vi "RT Subparse properties.vi"(5 "FIFO Index Decimation Table":i32[](array[numeric])=[0, 2, 2, 0, 3], 7 "Block Address decimation table":u32[](array[numeric])=[0, 2, 2, 0, 3], 8 "FIFO indexes":i32[](array[numeric])=[1, 2, 3, 4, 5], 9 "Block Address":u32[](array[numeric])=[0, 2, 2, 0, 3], 11 "Relative Address in Block":u32[](array[numeric])=[0, 0, 1, 5, 5]) -> (0 "error out":errorcluster, 2 "Array out":T1[](array[typedef]), 3 "max block size":u32)   [LabVIEW 2015, in "RefMem DMA Custom Device.lvlib"]
uses:
  RefMem DMA Custom Device.lvlib
  Block descriptor.ctl
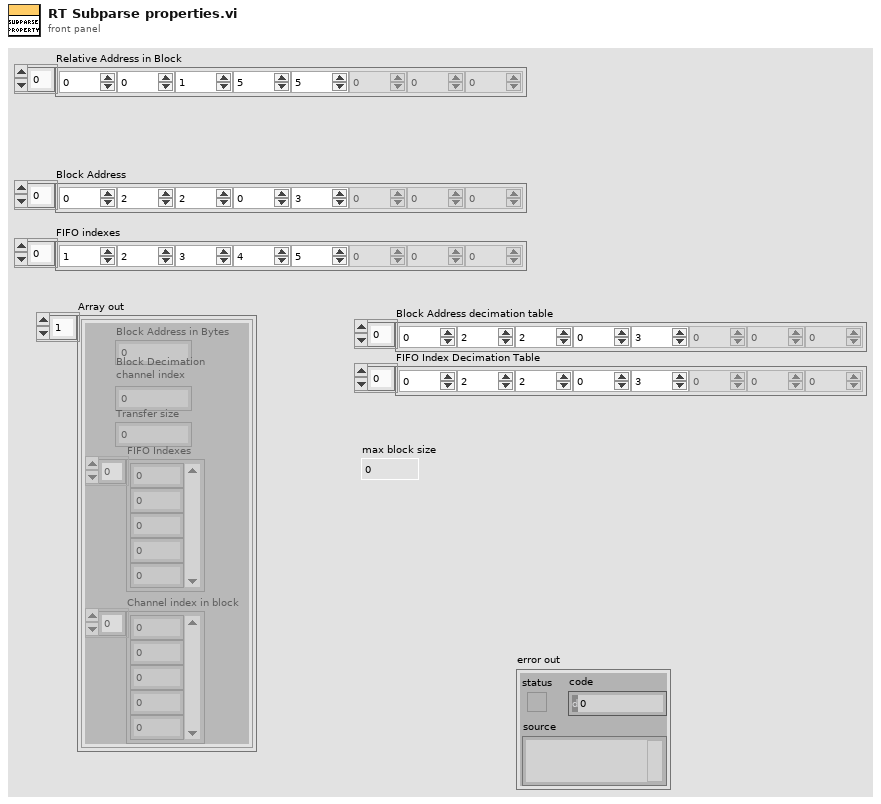
[diagram p1: front panel]
types:
  T1 = typedef "RefMem DMA Custom Device.lvlib/Block descriptor.ctl" = cluster{"Block Address in Bytes":u32, "Block Decimation \nchannel index":i32, "Transfer size":u32, "FIFO Indexes":i32[], "Channel index in block":i32[]}
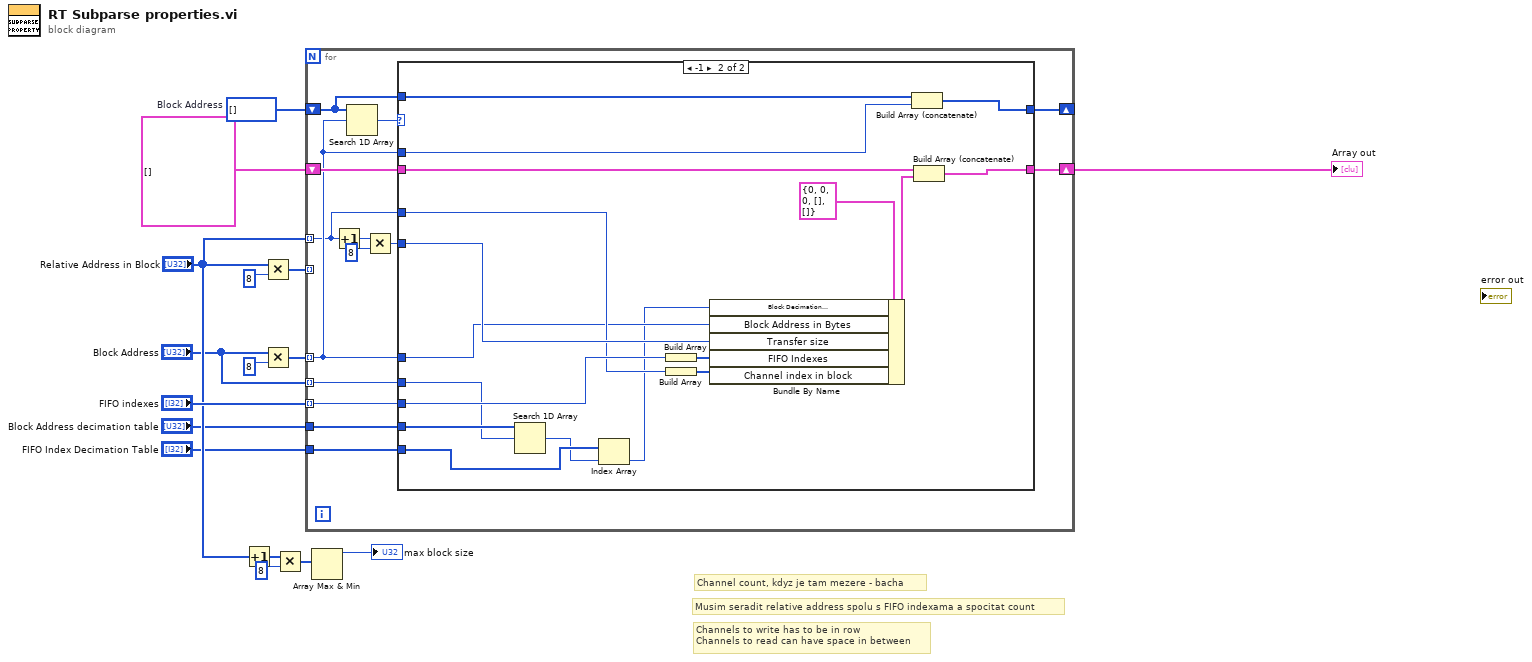
[diagram p0: block diagram]
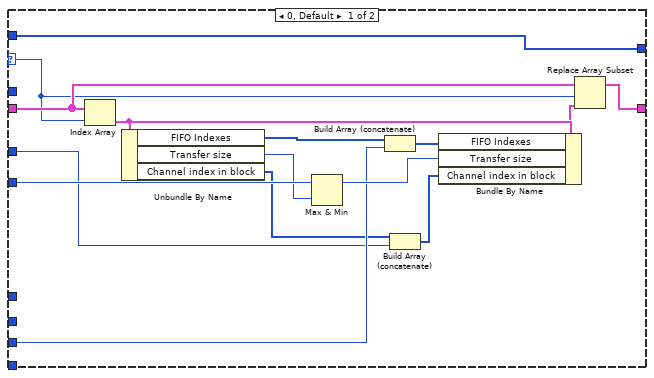
[diagram p2: hidden frame]
diagram:
  w15 = u32[] []  # Block Address
  # "Channel count, kdyz je tam mezere - bacha"
  # "Channels to write has to be in row\nChannels to read can have space in between"
  # "Musim seradit relative address spolu s FIFO indexama a spocitat count"
  n1 = Increment(x="Relative Address in Block") -> (x+1=w6:u32[])
  n2 = Multiply(x="Relative Address in Block", y=u32 8) -> (x*y=w11:u32[])
  n3 = Multiply(x="Block Address", y=u32 8) -> (x*y=w8:u32[])
  n4 = Multiply(x=w6, y=u32 8) -> (x*y=w4:u32[])
  n5 = for {
    tunnel: w8 -> [w25] mode=indexing
    tunnel: "FIFO indexes" -> [w24] mode=indexing
    shift-right: [w27] -> _
    shift-left: w15 -> [w29]
    shift-right: [w26] -> w13
    shift-left: T1[] [] ("Array out") -> [w28]
    tunnel: w11 -> [_] mode=indexing
    tunnel: "Relative Address in Block" -> [w20] mode=indexing
    tunnel: "Block Address decimation table" -> [w19]
    tunnel: "FIFO Index Decimation Table" -> [w18]
    tunnel: "Block Address" -> [w17] mode=indexing
    n6 = Increment(x=w20) -> (x+1=w23:u32)
    n7 = Search 1D Array(1D array=w29, element=w25) -> (index of element=w30:i32)  [unwired: 1 in]
    n8 = Multiply(x=w23, y=u32 8) -> (x*y=w21:u32)
    n9 = case shown="-1" w30 {
      selector: w30 -> [w43 _]
      tunnel: w29 -> [w40 w63]
      tunnel: w28 -> [w44 w62]
      tunnel: [w40 w61] -> w27
      tunnel: [w42 w60] -> w26
      tunnel: w25 -> [_ w59]
      tunnel: w25 -> [_ w50]
      tunnel: w24 -> [w34 w56]
      tunnel: w21 -> [w39 w54]
      tunnel: w20 -> [w31 w52]
      tunnel: w19 -> [_ w51]
      tunnel: w18 -> [_ w49]
      tunnel: w17 -> [_ w46]
      frame 0, Default {
        n10 = Index Array(array=w44, index=w43) -> (element=w45:T1)
        n11 = Unbundle By Name(w45) -> ("FIFO Indexes"=w36:i32[], "Transfer size"=w38:u32, "Channel index in block"=w32:i32[])
        n12 = Max & Min(x=w39, y=w38) -> (max(x,y)=w37:u32)  [unwired: 1 out]
        n13 = Build Array (concatenate)(w36, w34) -> (w35:i32[])
        n14 = Build Array (concatenate)(w32, w31) -> (w33:u32[])
        n15 = Bundle By Name(cluster=w45, "FIFO Indexes"=w35, "Transfer size"=w37, "Channel index in block"=w33) -> (w41:T1)
        n16 = Replace Array Subset(array=w44, new element=w41, index=w43) -> (w42:T1[])
      }
      frame -1 {
        n17 = Search 1D Array(1D array=w51, element=w46) -> (index of element=w48:i32)  [unwired: 1 in]
        n18 = Index Array(array=w49, index=w48) -> (element=w47:i32)
        n19 = Build Array(w56) -> (w55:i32[])
        n20 = Build Array(w52) -> (w53:u32[])
        n21 = Bundle By Name(cluster=T1 {"Block Address in Bytes"=0, "Block Decimation \nchannel index"=0, "Transfer size"=0, "FIFO Indexes"=[], "Channel index in block"=[]} ("Block descriptor"), "Block Decimation \nchannel index"=w47, "Block Address in Bytes"=w50, "Transfer size"=w54, "FIFO Indexes"=w55, "Channel index in block"=w53) -> (w57:T1)
        n22 = Build Array (concatenate)(w63, w59) -> (w61:u32[])
        n23 = Build Array (concatenate)(w62, w57) -> (w60:T1[])
      }
    }
  }
  "Array out" <- w13
  n24 = Array Max & Min(array=w4) -> (max value=→"max block size":u32)  [unwired: 3 out]
